vi "tarea 1.vi"() -> ()   [LabVIEW 2011]
panel:
  in  "stop":bool
  in  "Boolean 2":bool
  out "Boolean":bool
  out "Nivel Max":bool
  out "Nivel Medio":bool
  in  "Knob":i32(knob) scale=0.0..5.0
  out "tanque":i32(slide) scale=0.0..100.0
  # "El programa debera funcionar\nhasta que se presione el boton \nde detener.\nEl led se debe encender usando\nel boolean en la pc y en a protox\nlos niveles max y min se tiene que\nencender en la pc y en la protox.\n\nEl tanque se llena usando el knob\nque es una señal analogica.\n1 equivale a 20.\n\nMedio es 50\nMax es 80."
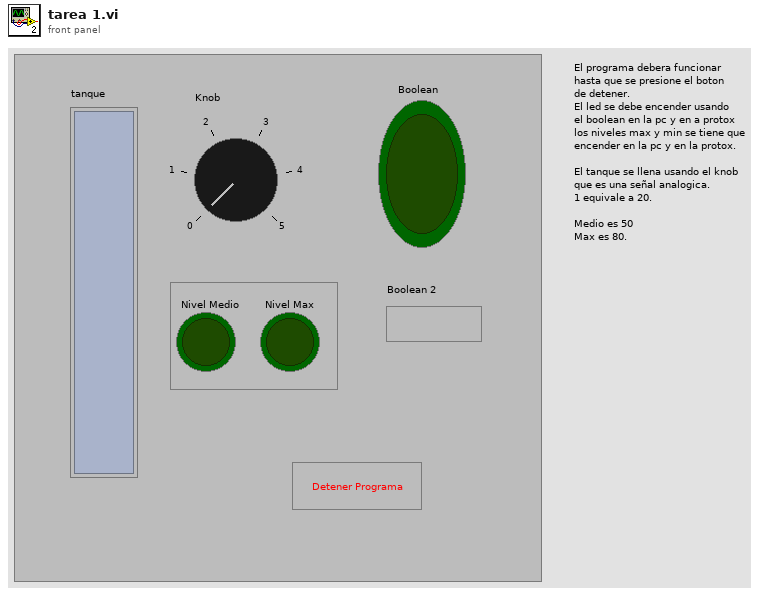
[diagram p1: front panel]
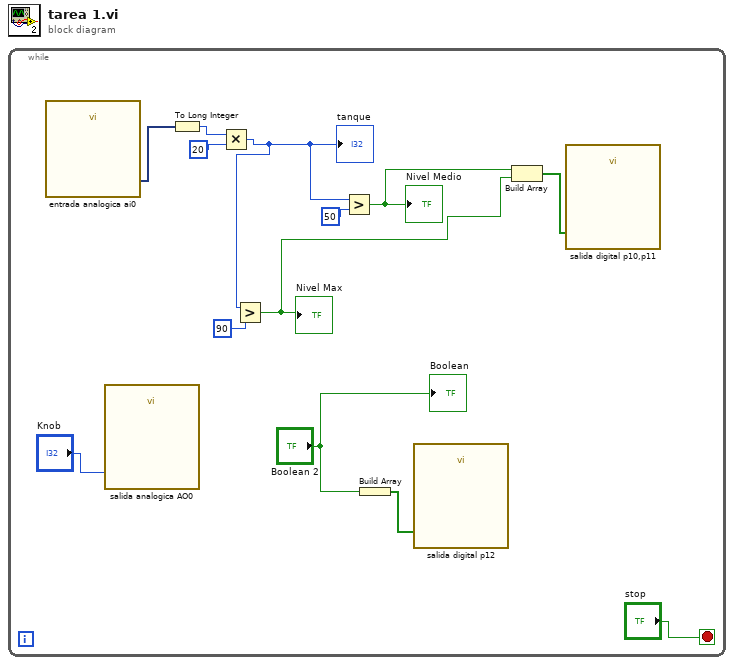
[diagram p0: block diagram]
diagram:
  n1 = while {
    stop <- "stop" stop-if-true
    n2 = call "entrada analogica ai0"() -> ("data"=w12:dynamicdata)  [unwired: 17 in, 2 out]
    n3 = call "salida analogica AO0"("data"="Knob") -> ()  [unwired: 17 in, 2 out]
    n4 = To Long Integer(number=w12) -> (32bit integer=w11:i32)
    n5 = Multiply(x=w11, y=20) -> (x*y=w6:i32)
    "tanque" <- w6
    n6 = Greater?(x=w6, y=90) -> (0:w5:bool)
    "Nivel Max" <- w5
    n7 = Greater?(x=w6, y=50) -> (0:w4:bool)
    "Nivel Medio" <- w4
    n8 = Build Array("Boolean 2") -> (w1:bool[])
    n9 = call "salida digital p12"("data"=w1) -> ()  [unwired: 17 in, 2 out]
    n10 = Build Array(w4, w5) -> (w3:bool[])
    n11 = call "salida digital p10,p11"("data"=w3) -> ()  [unwired: 17 in, 2 out]
    "Boolean" <- "Boolean 2"
  }
